vi "print board dll.vi"(7 "i":i32, 8 "error in (no error)":errorcluster, 9 "j":i32, 10 "k":i32, 11 "board":i8) -> (0 "error out":errorcluster, 3 "board out":i8)   [LabVIEW 2025, in "uncoverspace.lvlib"]
doc: "void print_board_dll(int8_t board[Z][Y][X], int k, int j, int i);\n\nvoid print_board_dll(int8_t *board, int k, int j, int i);"
uses:
  uncoverspace.lvlib
  uncoverspace.dll
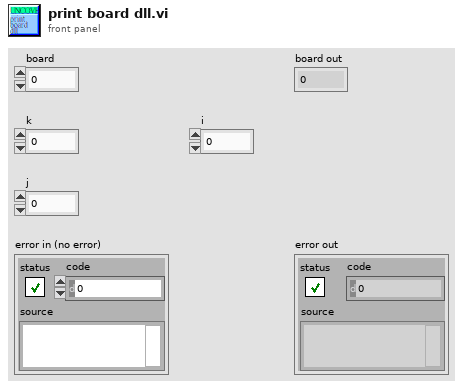
[diagram p1: front panel]
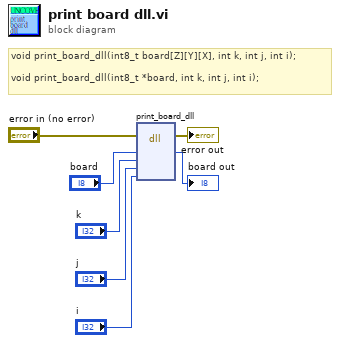
[diagram p0: block diagram]
diagram:
  # "void print_board_dll(int8_t board[Z][Y][X], int k, int j, int i);\n\nvoid print_board_dll(int8_t *board, int k, int j, int i);"
  n1 = dll-call lib="C:/Users/daimapi/Desktop/project/minesweeper/c_code/uncoverspace/uncoverspace.*" fn="print_board_dll"(error in="error in (no error)", "board"="board", "k"="k", "j"="j", "i"="i") -> (error out=→"error out":errorcluster, "board"=→"board out":i8)  [unwired: 6 in, 1 out]
